vi "SRDG535.ProcEvents.vi"(0 "i ref in":refnum<vi>, 5 "error in":errorcluster) -> (14 "i ref out":refnum<vi>, 19 "error out":errorcluster)   [LabVIEW 2014, in "SRDG535.lvlib"]
doc: "This method is used to define the events the object will listen to. Add your own events here."
uses:
  SRDG535.lvlib
  CSCore/BaseProcess/BaseProcess.event definition.ctl
  CSCore/CAEObj/CAEObj.event definition.ctl
  CSCore/BaseProcess/BaseProcess.descriptor string definition.ctl
  CSCore/BaseProcess/BaseProcess.lvlib
  CSCore/CAEObj/CAEObj.lvlib
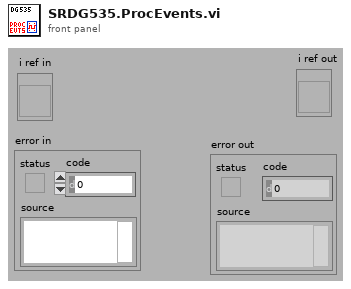
[diagram p1: front panel]
types:
  T1 = typedef "BaseProcess.lvlib/BaseProcess.event definition.ctl" = cluster{"CAEEvtDef":T2, "Data Descriptor":T3}
  T2 = typedef "CAEObj.lvlib/CAEObj.event definition.ctl" = cluster{"URL":string, "enable":bool, "ignoreResID":bool}
  T3 = typedef "BaseProcess.lvlib/BaseProcess.descriptor string definition.ctl" = string
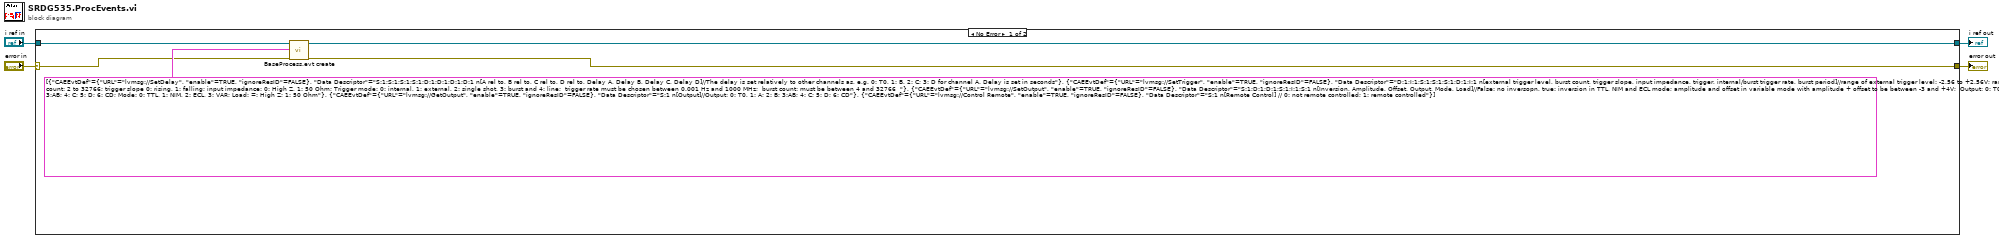
[diagram p0: block diagram]
diagram:
  n1 = case shown="No Error" "error in" {
    selector: "error in" -> [w5 w11]
    tunnel: "i ref in" -> [w9 w10]
    tunnel: [w8 w11] -> w3
    tunnel: [w7 w10] -> w2
    frame No Error {
      n2 = call "BaseProcess.evt create.vi"("i ref in"=w9, "newEvents"=T1[] [{"CAEEvtDef"={"URL"="lvmsg://SetDelay", "enable"=TRUE, "ignoreResID"=FALSE}, "Data Descriptor"="S:1;S:1;S:1;S:1;D:1;D:1;D:1;D:1 n[A rel to, B rel to, C rel to, D rel to, Delay A, Delay B, Delay C, Delay D]//The delay is set relatively to other channels as, e.g. 0: T0, 1: B, 2: C; 3: D for channel A. Delay is set in seconds"}, {"CAEEvtDef"={"URL"="lvmsg://SetTrigger", "enable"=TRUE, "ignoreResID"=FALSE}, "Data Descriptor"="D:1;I:1;S:1;S:1;S:1;D:1;I:1 n[external trigger level, burst count, trigger slope, input impedance, trigger, internal/burst trigger rate, burst period]//range of external trigger level: -2.56 to +2.56V; range of burst count: 2 to 32766; trigger slope 0: rising, 1: falling; input impedance: 0: High Z, 1: 50 Ohm; Trigger mode: 0: internal, 1: external, 2: single shot, 3: burst and 4: line;  trigger rate must be chosen between 0.001 Hz and 1000 MHz;  burst count: must be between 4 and 32766  "}, {"CAEEvtDef"={"URL"="lvmsg://SetOutput", "enable"=TRUE, "ignoreResID"=FALSE}, "Data Descriptor"="S:1;D:1;D:1;S:1;I:1;S:1 n[Inversion, Amplitude, Offset, Output, Mode, Load]//False: no inversopn, true: inversion in TTL, NIM and ECL mode; amplitude and offset in variable mode with amplitude + offset to be between -3 and +4V;  Output: 0: T0, 1: A; 2: B; 3:AB; 4: C; 5: D; 6: CD; Mode: 0: TTL, 1: NIM, 2: ECL, 3: VAR; Load: =: High Z; 1: 50 Ohm"}, {"CAEEvtDef"={"URL"="lvmsg://GetOutput", "enable"=TRUE, "ignoreResID"=FALSE}, "Data Descriptor"="S:1 n[Output]//Output: 0: T0, 1: A; 2: B; 3:AB; 4: C; 5: D; 6: CD"}, {"CAEEvtDef"={"URL"="lvmsg://Control Remote", "enable"=TRUE, "ignoreResID"=FALSE}, "Data Descriptor"="S:1 n[Remote Control] // 0: not remote controlled; 1: remote controlled"}] ("new events"), "error in (no error)"=w5) -> ("i ref out"=w7:refnum<vi>, "error out"=w8:errorcluster)  [unwired: 13 in, 2 out]
    }
    frame Error {
    }
  }
  "i ref out" <- w2
  "error out" <- w3
